vi "Pockels Cal-Highlight active file.vi"(8 "error in (no error)":errorcluster, 11 "ListBox in":refnum<vi>) -> (0 "error out":errorcluster)   [LabVIEW 2020]
uses:
  Globals/gl_Calibration globals.vi
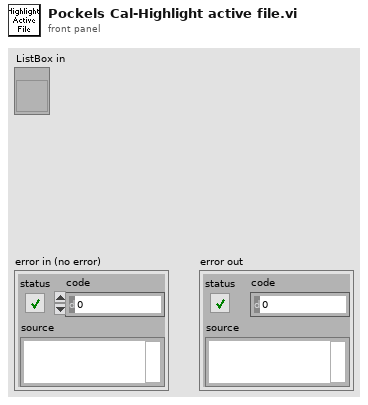
[diagram p1: front panel]
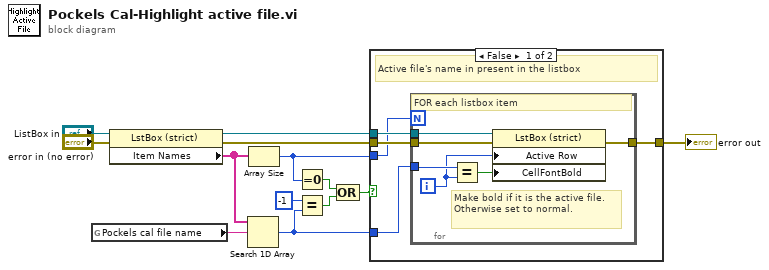
[diagram p0: block diagram]
diagram:
  n1 = global read "gl_Calibration globals.vi" "Pockels cal file name"() -> (w8:string)
  n2 = property on="Property Node" class="LstBox (strict)"(reference="ListBox in", error in="error in (no error)") -> (reference out=w9:refnum<vi>, error out=w10:errorcluster, "Item Names"=w7:string[])
  n3 = Search 1D Array(1D array=w7, element=w8) -> (index of element=w5:i32)  [unwired: 1 in]
  n4 = Array Size(array=w7) -> (size(s)=w6:i32)
  n5 = Equal To 0?(x=w6) -> (x = 0?=w3:bool)
  n6 = Equal?(x=-1, y=w5) -> (x = y?=w2:bool)
  n7 = Compound Arithmetic op=OR(w3, w2) -> (w1:bool)
  n8 = case shown="False" w1 {
    tunnel: [w18 w25] -> w12
    tunnel: w10 -> [w17 w25]
    tunnel: w9 -> [w16 _]
    tunnel: w6 -> [w15 _]
    tunnel: w5 -> [w14 _]
    frame False {
      # "Active file's name in present in the listbox"
      n9 = for {
        N: w15 -> [_]
        tunnel: [w24] -> w18
        tunnel: w17 -> [w23]
        tunnel: w16 -> [w22]
        tunnel: w14 -> [w21]
        i -> [w19]
        # "Make bold if it is the active file.\nOtherwise set to normal."
        # "FOR each listbox item"
        n10 = Equal?(x=w21, y=w19) -> (x = y?=w20:bool)
        n11 = property on="Property Node" class="LstBox (strict)"(reference=w22, error in=w23, "Active Row"=w19, "CellFontBold"=w20) -> (error out=w24:errorcluster)  [unwired: 1 out]
      }
    }
    frame True {
      # "Listbox is empty or active file's anme is not present"
    }
  }
  "error out" <- w12
